vi "Open By Index.vi"(7 "Enable Events (T)":bool=TRUE, 8 "Error In":errorcluster, 11 "Device Index":i32) -> (0 "Error Out":errorcluster, 2 "PS4 Event Refs":refnum<event-registration>, 3 "PS4 Controller Ref":T1)   [LabVIEW 2020, in "LMH-PS4.lvlib"]
doc: "Open a connection to the specified PS4 controller."
uses:
  LMH-PS4.lvlib
  Private/Type Defs/PS4 Controller Ref.ctl
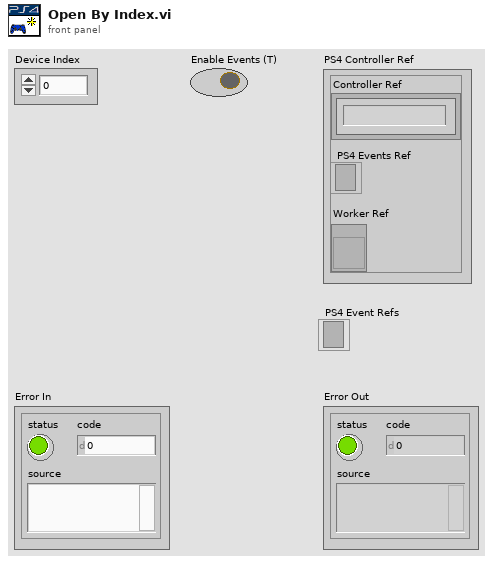
[diagram p1: front panel]
types:
  T1 = typedef "LMH-PS4.lvlib/PS4 Controller Ref.ctl" = cluster{"Controller Ref":refnum<k1>, "PS4 Events Ref":refnum<event-registration>, "Worker Ref":refnum<vi>}
  T2 = typedef "LMH-PS4.lvlib/PS4 Button Events.ctl" = cluster{"Square":refnum<user-event>, "X":refnum<user-event>, "Circle":refnum<user-event>, "Triangle":refnum<user-event>, "L1":refnum<user-event>, "R1":refnum<user-event>, "L2":refnum<user-event>, "R2":refnum<user-event>, "Share":refnum<user-event>, "Options":refnum<user-event>, "Left Thumbstick":refnum<user-event>, "Right Thumbstick":refnum<user-event>, "Playstation Button":refnum<user-event>, "Pad":refnum<user-event>}
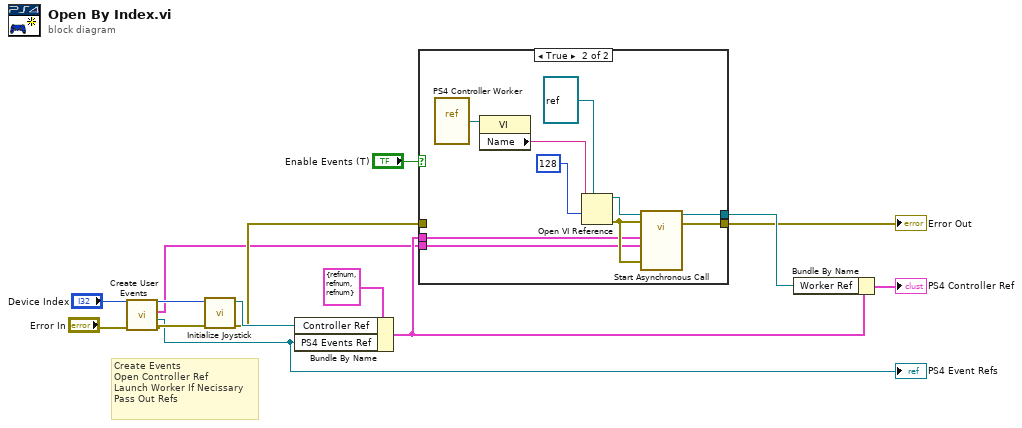
[diagram p0: block diagram]
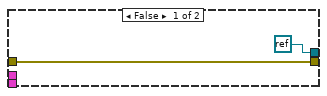
[diagram p2: hidden frame]
diagram:
  # "Create Events\nOpen Controller Ref\nLaunch Worker If Necissary\nPass Out Refs"
  n1 = call "Create User Events.vi"("Error In"="Error In") -> ("Error Out"=w5:errorcluster, "PS4 Event Refs"=w1:refnum<event-registration>, "Events"=w4:T2)  [unwired: 8 in]
  "PS4 Event Refs" <- w1
  n2 = call <vilib>:"Initialize Joystick.vi"("error in (no error)"=w5, "device index"="Device Index") -> ("error out"=w9:errorcluster, "device ID"=w10:refnum<k1>)  [unwired: 8 in]
  n3 = Bundle By Name(cluster=T1 {"Controller Ref"=refnum, "PS4 Events Ref"=refnum, "Worker Ref"=refnum} ("PS4 Controller Ref"), "Controller Ref"=w10, "PS4 Events Ref"=w1) -> (w11:T1)
  n4 = case shown="True" "Enable Events (T)" {
    tunnel: w4 -> [_ w18]
    tunnel: [refnum<k0> refnum w20] -> w12
    tunnel: w11 -> [_ w17]
    tunnel: [w14 w19] -> w8
    tunnel: w9 -> [w14 _]
    frame False {
    }
    frame True {
      n5 = vi-ref "PS4 Controller Worker.vi"() -> (w16:refnum<vi>)
      n6 = property class="VI"(reference=w16) -> ("Name"=w22:string)  [unwired: 1 in, 2 out]
      n7 = Open VI Reference(type specifier VI Refnum (for type only)=refnum<vi> refnum, vi path=w22, options=128) -> (vi reference=w23:refnum<vi>, error out=w21:errorcluster)  [unwired: 3 in]
      n8 = call-by-ref "Start Asynchronous Call"(reference=w23, error in=w21, "Error In 2"=w21, "PS4 Button Events"=w18, "PS4 Controller Ref"=w17) -> (reference out=w20:refnum<vi>, error out=w19:errorcluster)  [unwired: 8 in, 1 out]
    }
  }
  "Error Out" <- w8
  n9 = Bundle By Name(cluster=w11, "Worker Ref"=w12) -> (→"PS4 Controller Ref":T1)
